vi "Bohman Window (CDB).vi"(11 "X":cdb[](array[numeric])) -> (0 "error":i32, 3 "Windowed X":cdb[](array[numeric]))   [LabVIEW 2020, in "NI_AALPro.lvlib"]
doc: "Applies a Bohman window to the input signal <B>X</B>. Wire data to the <B>X</B> input to determine the polymorphic instance to use or manually select the instance."
uses:
  <vilib>/Analysis/NI_AALPro.lvlib
  <resource>/lvanlys.dll
panel:
  # "Bohman Window"
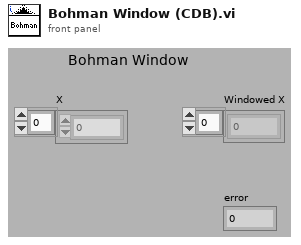
[diagram p1: front panel]
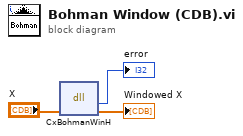
[diagram p0: block diagram]
diagram:
  n1 = dll-call lib="e:/builds/penguin/labview/branches/2020/dev/dist/resource/lvanlys.*" fn="CxBohmanWinH"("X"="X") -> ("error"=→"error":i32, "X"=→"Windowed X":cdb[])  [unwired: 3 in, 2 out]
